vi "filter.filter.add.vi"(11 "filter.data in":T1 {"get.state"."v"."Quantity" format="%.0x"; "get.state"."v"."OrderId" format="%.0x"; "mem.cmd"."ord.2"."v"."Quantity" format="%016x"; "mem.cmd"."ord.2"."v"."OrderId" format="%016x"; "mem.cmd"."ord.1"."v"."Quantity" format="%016x"; "mem.cmd"."ord.1"."v"."OrderId" format="%016x"; "mem.cmd"."ticker"."v"."Symbol" format="%016x"; "mem.cmd"."order.slot.value"."Quantity" format="%016x"; "mem.cmd"."order.slot.value"."OrderId" format="%016x"; "debug"."v"."slot.3" format="%.0x"; "debug"."v"."slot.2" format="%.0x"; "debug"."v"."slot.1" format="%.0x"; "debug"."v"."slot.0" format="%.0x"; "Scratch"."OrderId" format="%016x"; "hash.2"."data.in" format="%.0x"; "hash.2"."crc32.out" format="%.0x"; "hash.1"."data.in" format="%.0x"; "hash.1"."crc32.out" format="%.0x"}) -> (3 "filter.data out":T1 {"get.state"."v"."Quantity" format="%.0x"; "get.state"."v"."OrderId" format="%.0x"; "mem.cmd"."ord.2"."v"."Quantity" format="%016x"; "mem.cmd"."ord.2"."v"."OrderId" format="%016x"; "mem.cmd"."ord.1"."v"."Quantity" format="%016x"; "mem.cmd"."ord.1"."v"."OrderId" format="%016x"; "mem.cmd"."ticker"."v"."Symbol" format="%016x"; "mem.cmd"."order.slot.value"."Quantity" format="%016x"; "mem.cmd"."order.slot.value"."OrderId" format="%016x"; "debug"."v"."slot.3" format="%.0x"; "debug"."v"."slot.2" format="%.0x"; "debug"."v"."slot.1" format="%.0x"; "debug"."v"."slot.0" format="%.0x"; "Scratch"."OrderId" format="%016x"; "hash.2"."data.in" format="%.0x"; "hash.2"."crc32.out" format="%.0x"; "hash.1"."data.in" format="%.0x"; "hash.1"."crc32.out" format="%.0x"})   [LabVIEW 2020]
uses:
  order.slot.ctl
  ticker.slot.ctl
  filter.memory.command.ctl
  filter.states.ctl
  filter.debug.slot.ctl
  filter.debug.ctl
  order.slot.hm.ctl
  order.slot.access.ctl
  ticker.slot.access.ctl
  filter.data.scratch.ctl
  filter.data.ctl
  Market.Data.Common/fpga/orderbook.command.ctl
  Market.Data.Common/fpga/fpganow.common.fpga.lvlib
  filter.state.slot.ctl
  filter.state.ctl
  Market.Data.Common/fpga/orderbook.command.type.ctl
  filter.hash.ctl
  Filter.lvclass
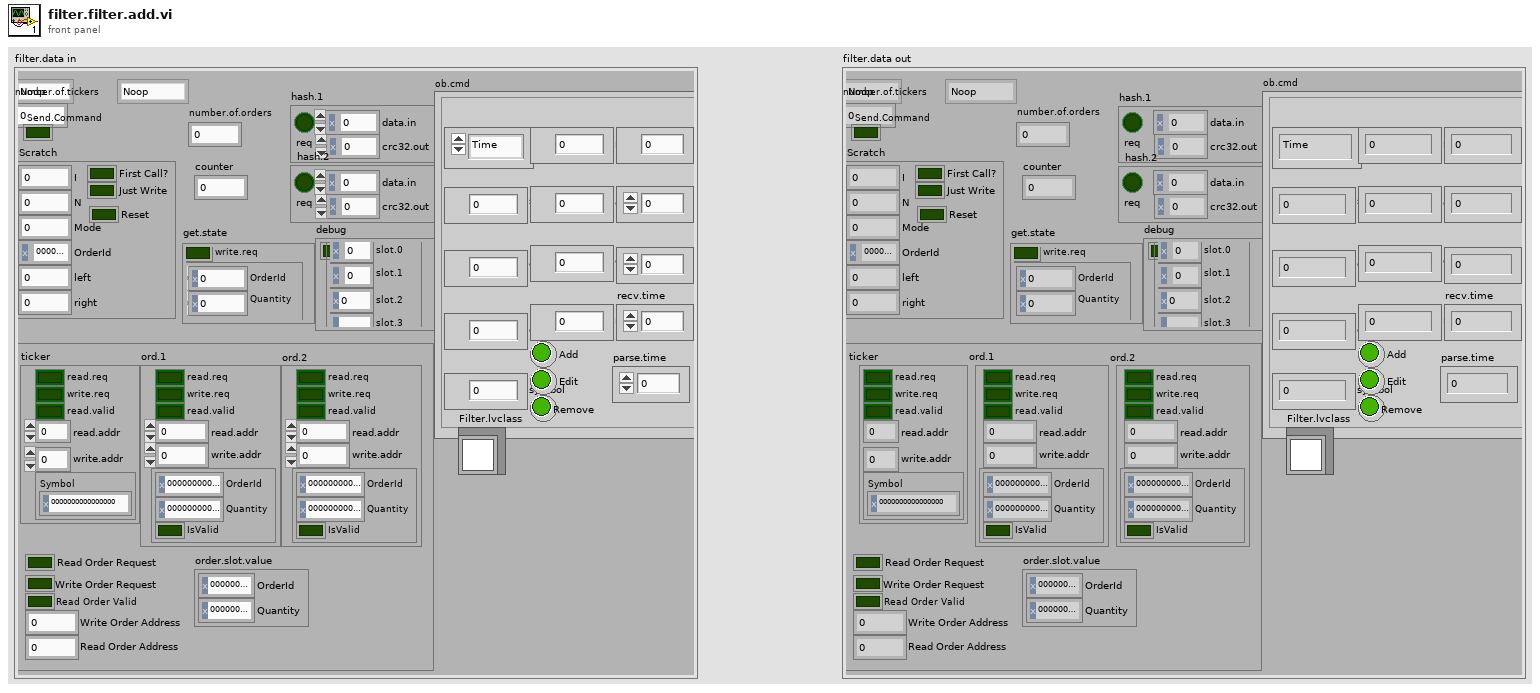
[diagram p1: front panel]
types:
  T1 = typedef "filter.data.ctl" = cluster{"filter.state":T2, "number.of.tickers":u32, "filter.saved.state":T2, "Send.Command":bool, "hash.1":T3, "hash.2":T3, "Scratch":T4, "debug":T5, "mem.cmd":T7, "get.state":T13, "ob.cmd":T15, "number.of.orders":u32, "Filter.lvclass":refnum<class "Filter.lvclass">, "counter":i16}
  T2 = typedef "filter.states.ctl" = enum16{"Noop", "Reset", "Debug", "Configuration", "Wait.for.Command", "Filter.Add", "Filter.Other", "Insert.Order", "Delete Order", "Get.State", "Get.Watchlist", "Get.Memory"}
  T3 = typedef "filter.hash.ctl" = cluster{"req":bool, "data.in":u64, "crc32.out":u32}
  T4 = typedef "filter.data.scratch.ctl" = cluster{"I":u32, "N":u32, "Mode":u32, "OrderId":u64, "First Call?":bool, "Just Write":bool, "left":u32, "right":u32, "Reset":bool}
  T5 = typedef "filter.debug.ctl" = cluster{"write":bool, "v":T6}
  T6 = typedef "filter.debug.slot.ctl" = cluster{"slot.0":u64, "slot.1":u64, "slot.2":u64, "slot.3":u64}
  T7 = typedef "filter.memory.command.ctl" = cluster{"Read Order Request":bool, "Write Order Request":bool, "Read Order Valid":bool, "Write Order Address":u32, "Read Order Address":u32, "order.slot.value":T8, "ticker":T9, "ord.1":T11, "ord.2":T11}
  T8 = typedef "order.slot.ctl" = cluster{"OrderId":u64, "Quantity":u64}
  T9 = typedef "ticker.slot.access.ctl" = cluster{"read.req":bool, "write.req":bool, "read.valid":bool, "read.addr":u32, "write.addr":u32, "v":T10}
  T10 = typedef "ticker.slot.ctl" = cluster{"Symbol":u64}
  T11 = typedef "order.slot.access.ctl" = cluster{"read.req":bool, "write.req":bool, "read.valid":bool, "read.addr":u32, "write.addr":u32, "v":T12}
  T12 = typedef "order.slot.hm.ctl" = cluster{"OrderId":u64, "Quantity":u64, "IsValid":bool}
  T13 = typedef "filter.state.ctl" = cluster{"write.req":bool, "v":T14}
  T14 = typedef "filter.state.slot.ctl" = cluster{"OrderId":u64, "Quantity":u64}
  T15 = typedef "fpganow.common.fpga.lvlib/orderbook.command.ctl" = cluster{"type":T16, "side":u8, "orderId ":u64, "quantity":u32, "symbol":u64, "price":u64, "executed.qty":u32, "canceled.qty":u32, "remaining.qty":u32, "seconds":u64, "nanoseconds":u64, "Add":bool, "Edit":bool, "Remove":bool, "seq no":u32, "recv.time":u64, "parse.time":u64}
  T16 = typedef "fpganow.common.fpga.lvlib/orderbook.command.type.ctl" = enum8{"Time", "AddOrder", "OrderExecuted", "OrderExecutedAtPrice", "ReduceSize", "ModifyOrder", "DeleteOrder", "Get.Everything", "Get.All.Orders", "Get.Top"}
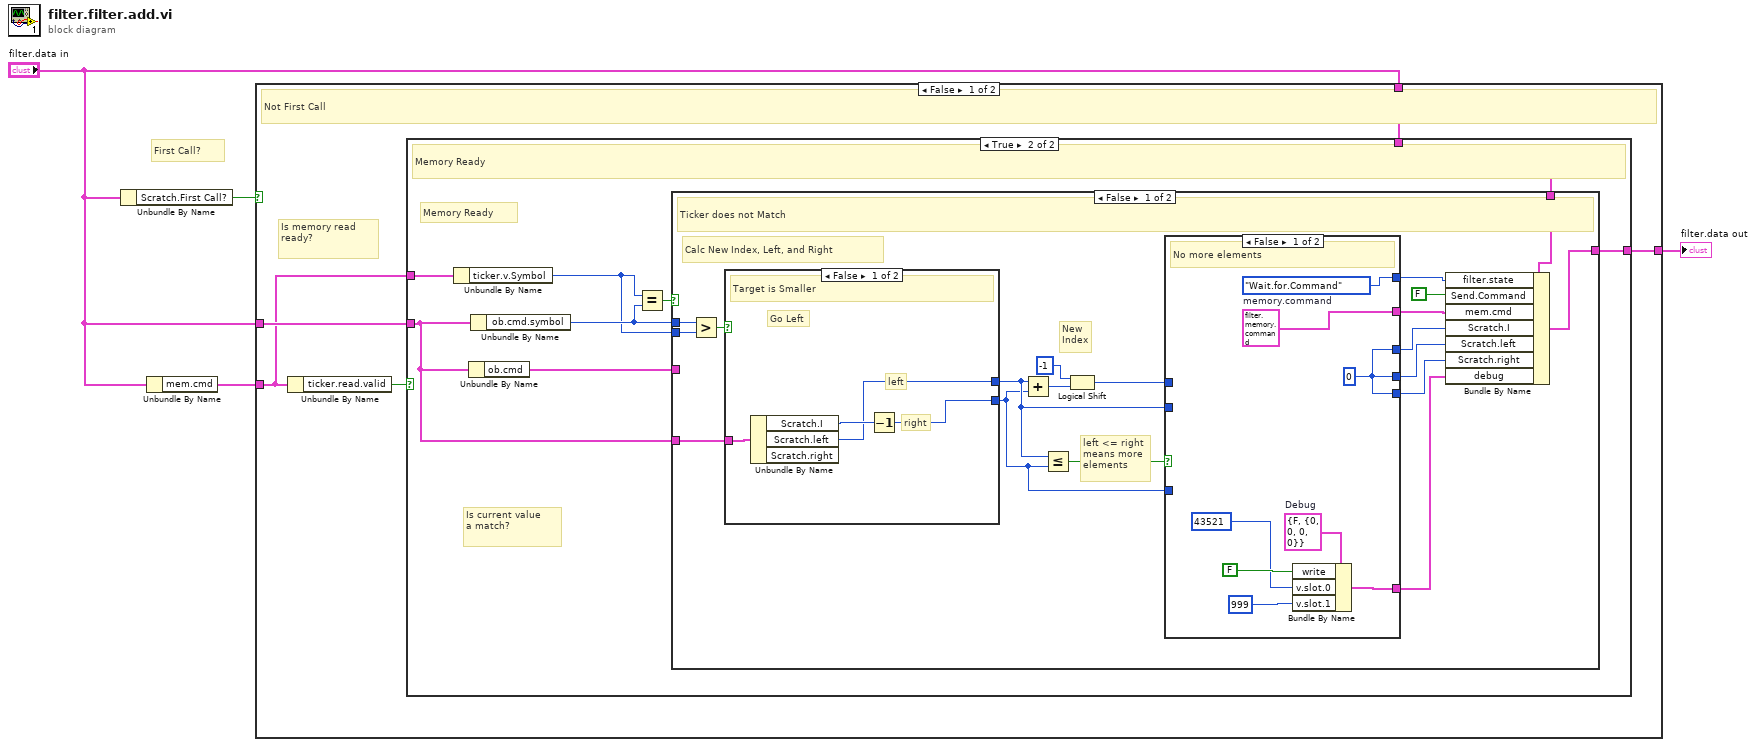
[diagram p0: block diagram]
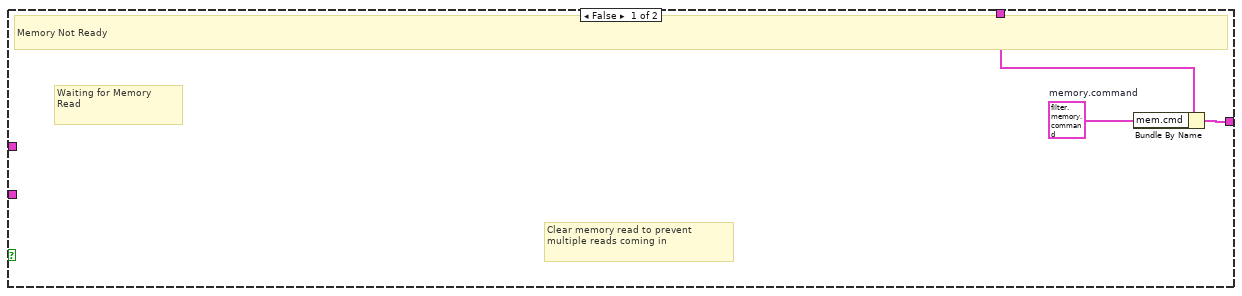
[diagram p2: hidden frame]
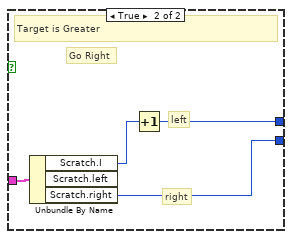
[diagram p3: hidden frame]
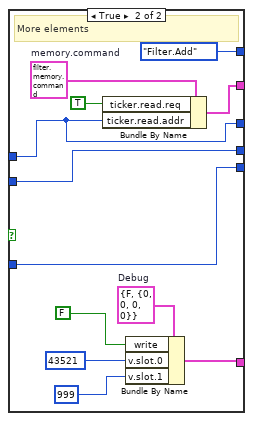
[diagram p4: hidden frame]
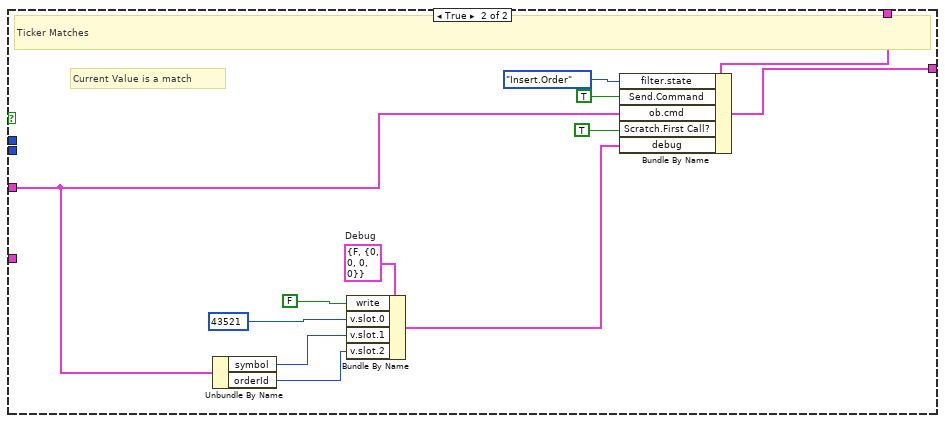
[diagram p5: hidden frame]
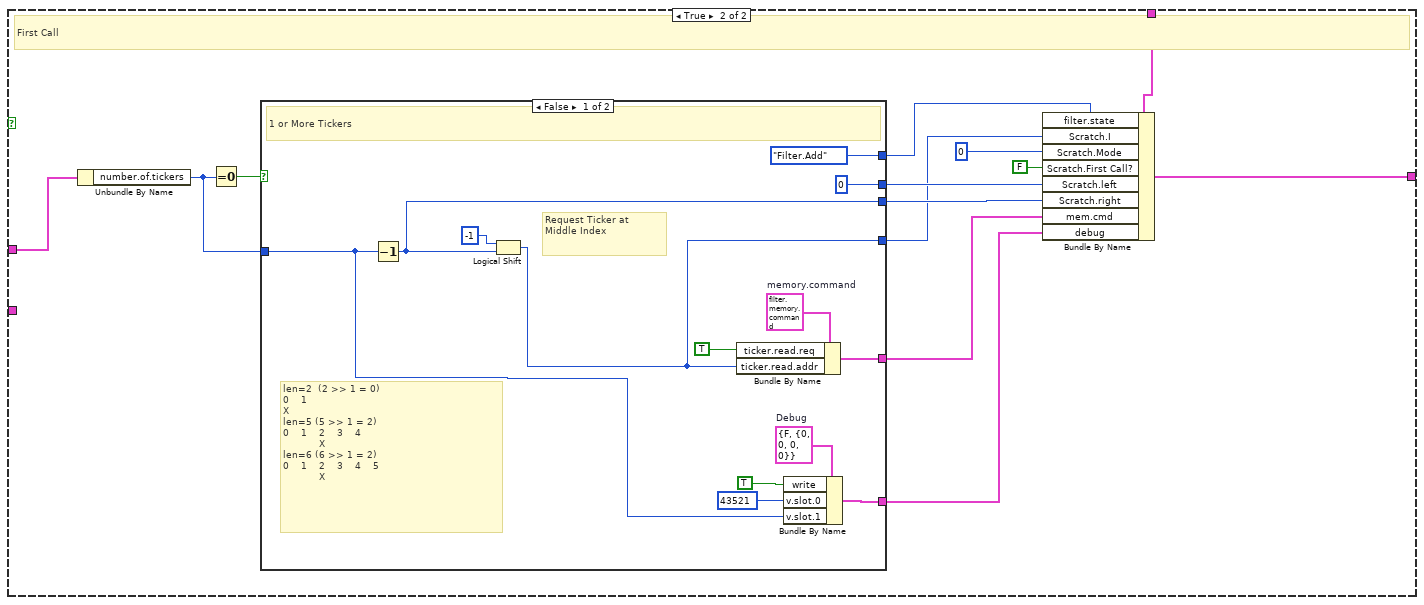
[diagram p6: hidden frame]
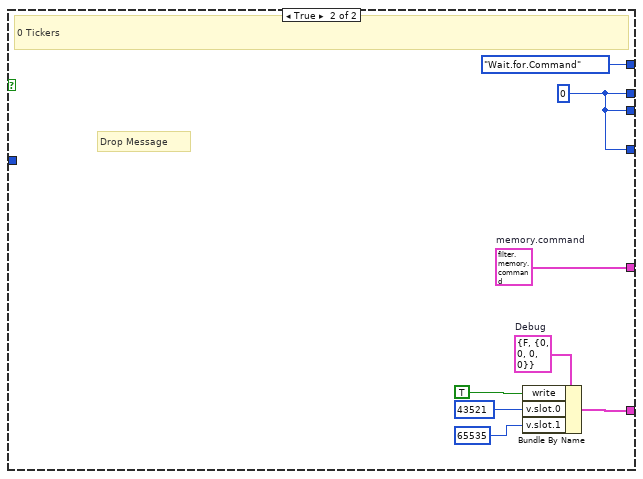
[diagram p7: hidden frame]
diagram:
  # "First Call?"
  n1 = Unbundle By Name("filter.data in") -> ("Scratch.First Call?"=w1:bool)
  n2 = Unbundle By Name("filter.data in") -> ("mem.cmd"=w3:T7)
  n3 = case shown="False" w1 {
    tunnel: "filter.data in" -> [w7 w92]
    tunnel: [w8 w91] -> w2
    tunnel: w3 -> [w5 _]
    tunnel: "filter.data in" -> [w6 w87]
    frame False {
      # "Is memory read\nready?"
      # "Not First Call"
      n4 = Unbundle By Name(w5) -> ("ticker.read.valid"=w9:bool)
      n5 = case shown="True" w9 {
        tunnel: [w10 w17] -> w8
        tunnel: w7 -> [w12 w18]
        tunnel: w6 -> [_ w15]
        tunnel: w5 -> [_ w20]
        frame False {
          w11 = T7 {"Read Order Request"=FALSE, "Write Order Request"=FALSE, "Read Order Valid"=FALSE, "Write Order Address"=0, "Read Order Address"=0, "order.slot.value"={"OrderId"=0, "Quantity"=0}, "ticker"={"read.req"=FALSE, "write.req"=FALSE, "read.valid"=FALSE, "read.addr"=0, "write.addr"=0, "v"={"Symbol"=0}}, "ord.1"={"read.req"=FALSE, "write.req"=FALSE, "read.valid"=FALSE, "read.addr"=0, "write.addr"=0, "v"={"OrderId"=0, "Quantity"=0, "IsValid"=FALSE}}, "ord.2"={"read.req"=FALSE, "write.req"=FALSE, "read.valid"=FALSE, "read.addr"=0, "write.addr"=0, "v"={"OrderId"=0, "Quantity"=0, "IsValid"=FALSE}}}  # memory.command
          # "Clear memory read to prevent\nmultiple reads coming in"
          # "Waiting for Memory\nRead"
          # "Memory Not Ready"
          n6 = Bundle By Name(cluster=w12, "mem.cmd"=w11) -> (w10:T1)
        }
        frame True {
          # "Is current value\na match?"
          # "Memory Ready"
          # "Memory Ready"
          n7 = Unbundle By Name(w20) -> ("ticker.v.Symbol"=w13:u64)
          n8 = Unbundle By Name(w15) -> ("ob.cmd"=w16:T15)
          n9 = Unbundle By Name(w15) -> ("ob.cmd.symbol"=w14:u64)
          n10 = Equal?(x=w13, y=w14) -> (x = y?=w19:bool)
          n11 = case shown="False" w19 {
            tunnel: w18 -> [w38 w79]
            tunnel: [w39 w77] -> w17
            tunnel: w16 -> [_ w71]
            tunnel: w15 -> [w29 _]
            tunnel: w14 -> [w32 _]
            tunnel: w13 -> [w31 _]
            frame False {
              # "left <= right\nmeans more\nelements"
              # "New\nIndex"
              # "Calc New Index, Left, and Right"
              # "Ticker does not Match"
              n12 = Greater?(x=w32, y=w31) -> (0:w30:bool)
              n13 = case shown="False" w30 {
                tunnel: w29 -> [w42 w47]
                tunnel: [w41 w45] -> w23
                tunnel: [w40 w44] -> w22
                frame False {
                  # "right"
                  # "left"
                  # "Go Left"
                  # "Target is Smaller"
                  n14 = Unbundle By Name(w42) -> ("Scratch.I"=w43:u32, "Scratch.left"=w41:u32)  [unwired: 1 out]
                  n15 = Decrement(x=w43) -> (x-1=w40:u32)
                }
                frame True {
                  # "right"
                  # "left"
                  # "Go Right"
                  # "Target is Greater"
                  n16 = Unbundle By Name(w47) -> ("Scratch.I"=w46:u32, "Scratch.right"=w44:u32)  [unwired: 1 out]
                  n17 = Increment(x=w46) -> (x+1=w45:u32)
                }
              }
              n18 = Add(x=w23, y=w22) -> (x+y=w27:u32)
              n19 = Less Or Equal?(x=w23, y=w22) -> (x <= y?=w26:bool)
              n20 = Logical Shift(y=i16 -1, x=w27) -> (x << y=w25:u32)
              n21 = case shown="False" w26 {
                tunnel: [w54 w65] -> w37
                tunnel: [filter.states."Wait.for.Command" ("filter.state") filter.states."Filter.Add" ("filter.state")] -> w36
                tunnel: [w49 w63] -> w34
                tunnel: [w51 w56] -> w33
                tunnel: w25 -> [_ w63]
                tunnel: [w49 w62] -> w24
                tunnel: w23 -> [_ w62]
                tunnel: w22 -> [_ w61]
                tunnel: [w49 w61] -> w21
                frame False {
                  w53 = T5 {"write"=FALSE, "v"={"slot.0"=0, "slot.1"=0, "slot.2"=0, "slot.3"=0}}  # Debug
                  w49 = u32 0
                  w54 = T7 {"Read Order Request"=FALSE, "Write Order Request"=FALSE, "Read Order Valid"=FALSE, "Write Order Address"=0, "Read Order Address"=0, "order.slot.value"={"OrderId"=0, "Quantity"=0}, "ticker"={"read.req"=FALSE, "write.req"=FALSE, "read.valid"=FALSE, "read.addr"=0, "write.addr"=0, "v"={"Symbol"=0}}, "ord.1"={"read.req"=FALSE, "write.req"=FALSE, "read.valid"=FALSE, "read.addr"=0, "write.addr"=0, "v"={"OrderId"=0, "Quantity"=0, "IsValid"=FALSE}}, "ord.2"={"read.req"=FALSE, "write.req"=FALSE, "read.valid"=FALSE, "read.addr"=0, "write.addr"=0, "v"={"OrderId"=0, "Quantity"=0, "IsValid"=FALSE}}}  # memory.command
                  # "No more elements"
                  n22 = Bundle By Name(cluster=w53, "write"=FALSE ("Write.to.Debug"), "v.slot.0"=u64 43521 ("debug.slot.Ticker"), "v.slot.1"=u64 999 ("debug.slot.OrderId")) -> (w51:T5)
                }
                frame True {
                  w60 = T5 {"write"=FALSE, "v"={"slot.0"=0, "slot.1"=0, "slot.2"=0, "slot.3"=0}}  # Debug
                  w67 = T7 {"Read Order Request"=FALSE, "Write Order Request"=FALSE, "Read Order Valid"=FALSE, "Write Order Address"=0, "Read Order Address"=0, "order.slot.value"={"OrderId"=0, "Quantity"=0}, "ticker"={"read.req"=FALSE, "write.req"=FALSE, "read.valid"=FALSE, "read.addr"=0, "write.addr"=0, "v"={"Symbol"=0}}, "ord.1"={"read.req"=FALSE, "write.req"=FALSE, "read.valid"=FALSE, "read.addr"=0, "write.addr"=0, "v"={"OrderId"=0, "Quantity"=0, "IsValid"=FALSE}}, "ord.2"={"read.req"=FALSE, "write.req"=FALSE, "read.valid"=FALSE, "read.addr"=0, "write.addr"=0, "v"={"OrderId"=0, "Quantity"=0, "IsValid"=FALSE}}}  # memory.command
                  # "More elements"
                  n23 = Bundle By Name(cluster=w67, "ticker.read.req"=TRUE ("ticker.slot"), "ticker.read.addr"=w63) -> (w65:T7)
                  n24 = Bundle By Name(cluster=w60, "write"=FALSE ("Write.to.Debug"), "v.slot.0"=u64 43521 ("debug.slot.Ticker"), "v.slot.1"=u64 999 ("debug.slot.OrderId")) -> (w56:T5)
                }
              }
              n25 = Bundle By Name(cluster=w38, "filter.state"=w36, "Send.Command"=FALSE, "mem.cmd"=w37, "Scratch.I"=w34, "Scratch.left"=w24, "Scratch.right"=w21, "debug"=w33) -> (w39:T1)
            }
            frame True {
              w74 = T5 {"write"=FALSE, "v"={"slot.0"=0, "slot.1"=0, "slot.2"=0, "slot.3"=0}}  # Debug
              # "Current Value is a match"
              # "Ticker Matches"
              n26 = Unbundle By Name(w71) -> ("symbol"=w69:u64, "orderId"=w68:u64)
              n27 = Bundle By Name(cluster=w74, "write"=FALSE ("Write.to.Debug"), "v.slot.0"=u64 43521, "v.slot.1"=w69, "v.slot.2"=w68) -> (w72:T5)
              n28 = Bundle By Name(cluster=w79, "filter.state"=filter.states."Insert.Order", "Send.Command"=TRUE, "ob.cmd"=w71, "Scratch.First Call?"=TRUE, "debug"=w72) -> (w77:T1)
            }
          }
        }
      }
    }
    frame True {
      # "First Call"
      n29 = Unbundle By Name(w87) -> ("number.of.tickers"=w81:u32)
      n30 = Equal To 0?(x=w81) -> (x = 0?=w88:bool)
      n31 = case shown="False" w88 {
        tunnel: [w103 w112] -> w84
        tunnel: [filter.states."Filter.Add" ("filter.state") filter.states."Wait.for.Command" ("filter.state")] -> w86
        tunnel: [w99 w109] -> w85
        tunnel: [u32 0 ("Scratch.left") w106] -> w83
        tunnel: [w96 w106] -> w82
        tunnel: w81 -> [w93 _]
        tunnel: [w95 w106] -> w80
        frame False {
          w101 = T5 {"write"=FALSE, "v"={"slot.0"=0, "slot.1"=0, "slot.2"=0, "slot.3"=0}}  # Debug
          w105 = T7 {"Read Order Request"=FALSE, "Write Order Request"=FALSE, "Read Order Valid"=FALSE, "Write Order Address"=0, "Read Order Address"=0, "order.slot.value"={"OrderId"=0, "Quantity"=0}, "ticker"={"read.req"=FALSE, "write.req"=FALSE, "read.valid"=FALSE, "read.addr"=0, "write.addr"=0, "v"={"Symbol"=0}}, "ord.1"={"read.req"=FALSE, "write.req"=FALSE, "read.valid"=FALSE, "read.addr"=0, "write.addr"=0, "v"={"OrderId"=0, "Quantity"=0, "IsValid"=FALSE}}, "ord.2"={"read.req"=FALSE, "write.req"=FALSE, "read.valid"=FALSE, "read.addr"=0, "write.addr"=0, "v"={"OrderId"=0, "Quantity"=0, "IsValid"=FALSE}}}  # memory.command
          # "len=2  (2 >> 1 = 0)\n0    1\nX\nlen=5 (5 >> 1 = 2)\n0    1    2    3    4 \n            X\nlen=6 (6 >> 1 = 2)\n0    1    2    3    4    5\n            X"
          # "Request Ticker at\nMiddle Index"
          # "1 or More Tickers"
          n32 = Decrement(x=w93) -> (x-1=w96:u32)
          n33 = Logical Shift(y=i16 -1, x=w96) -> (x << y=w95:u32)
          n34 = Bundle By Name(cluster=w105, "ticker.read.req"=TRUE ("ticker.slot"), "ticker.read.addr"=w95) -> (w103:T7)
          n35 = Bundle By Name(cluster=w101, "write"=TRUE ("Write.to.Debug"), "v.slot.0"=u64 43521 ("Ticker"), "v.slot.1"=w93) -> (w99:T5)
        }
        frame True {
          w106 = u32 0 ("Scratch.left")
          w111 = T5 {"write"=FALSE, "v"={"slot.0"=0, "slot.1"=0, "slot.2"=0, "slot.3"=0}}  # Debug
          w112 = T7 {"Read Order Request"=FALSE, "Write Order Request"=FALSE, "Read Order Valid"=FALSE, "Write Order Address"=0, "Read Order Address"=0, "order.slot.value"={"OrderId"=0, "Quantity"=0}, "ticker"={"read.req"=FALSE, "write.req"=FALSE, "read.valid"=FALSE, "read.addr"=0, "write.addr"=0, "v"={"Symbol"=0}}, "ord.1"={"read.req"=FALSE, "write.req"=FALSE, "read.valid"=FALSE, "read.addr"=0, "write.addr"=0, "v"={"OrderId"=0, "Quantity"=0, "IsValid"=FALSE}}, "ord.2"={"read.req"=FALSE, "write.req"=FALSE, "read.valid"=FALSE, "read.addr"=0, "write.addr"=0, "v"={"OrderId"=0, "Quantity"=0, "IsValid"=FALSE}}}  # memory.command
          # "Drop Message"
          # "0 Tickers"
          n36 = Bundle By Name(cluster=w111, "write"=TRUE ("Write.to.Debug"), "v.slot.0"=u64 43521 ("debug.slot.Ticker"), "v.slot.1"=u64 65535 ("debug.slot.OrderId")) -> (w109:T5)
        }
      }
      n37 = Bundle By Name(cluster=w92, "filter.state"=w86, "Scratch.I"=w80, "Scratch.Mode"=u32 0, "Scratch.First Call?"=FALSE, "Scratch.left"=w83, "Scratch.right"=w82, "mem.cmd"=w84, "debug"=w85) -> (w91:T1)
    }
  }
  "filter.data out" <- w2
